vi "play_sound.vi"(7 "error in":errorcluster, 9 "Data":dynamicdata(waveform), 10 "Device":u32) -> (0 "error out":errorcluster)   [LabVIEW 2019]
doc: "Plays data from the sound output device using finite sampling. This Express VI automatically configures an output task and clears the task after the output completes.\n--------------------\n\nThis Express VI is configured as follows:\n\nDevice: 0"
panel:
  in  "Timeout (sec)":dbl=-1.0
  in  "Path":path
  in  "Use rate":bool
  in  "Sample rate (Hz)":dbl=22050.0
  in  "Resolution (bits)":i32=16
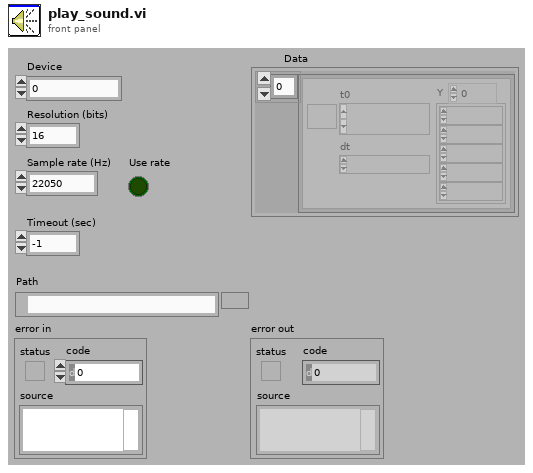
[diagram p1: front panel]
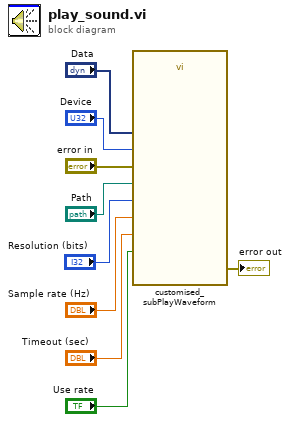
[diagram p0: block diagram]
diagram:
  n1 = call "customised_subPlayWaveform.vi"("Device"="Device", "Resolution (bits)"="Resolution (bits)", "Sample rate (Hz)"="Sample rate (Hz)", "Use rate"="Use rate", "Path"="Path", "error in (no error)"="error in", "Data"="Data", "Timeout (sec)"="Timeout (sec)") -> ("error out"=→"error out":errorcluster)  [unwired: 11 in]
